vi "Is New State.vi"(8 "error in (no error)":errorcluster, 11 "Command in":refnum<class "Command.lvclass">) -> (0 "error out":errorcluster, 3 "Command out":refnum<class "Command.lvclass">)   [LabVIEW 2013, in "Command.lvclass"]
uses:
  Command.lvclass
  Command.lvclass/Command.ctl
  States/State/State.lvclass
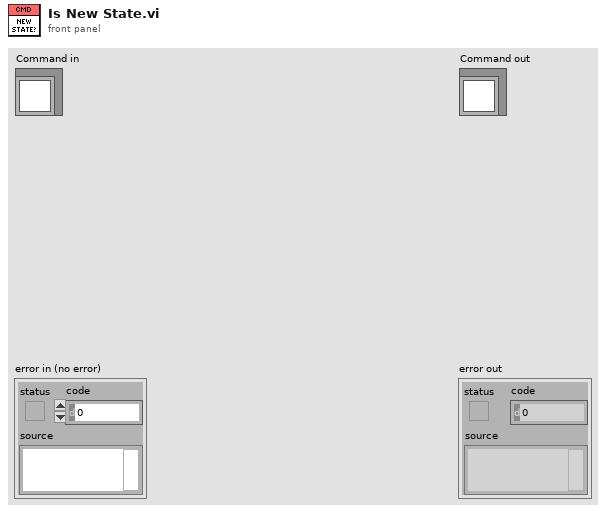
[diagram p1: front panel]
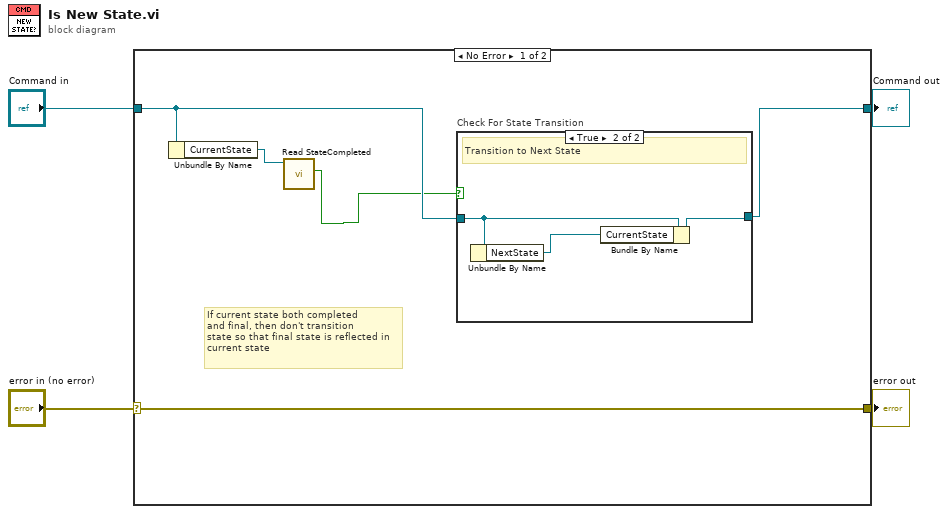
[diagram p0: block diagram]
diagram:
  n1 = case shown="No Error" "error in (no error)" {
    selector: "error in (no error)" -> [w9 w15]
    tunnel: [w9 w15] -> w3
    tunnel: [w6 w14] -> w1
    tunnel: "Command in" -> [w7 w14]
    frame No Error {
      # "If current state both completed\nand final, then don't transition \nstate so that final state is reflected in \ncurrent state"
      n2 = Unbundle By Name(w7) -> ("CurrentState"=w8:refnum<class "State.lvclass">)
      n3 = call-dynamic "Read StateCompleted.vi"("State in"=w8) -> ("StateCompleted"=w5:bool)  [unwired: 8 in, 2 out]
      n4 = case "Check For State Transition" shown="True" w5 {
        tunnel: [w10 w12] -> w6
        tunnel: w7 -> [w10 w13]
        frame False {
          # "No State Transition"
        }
        frame True {
          # "Transition to Next State"
          n5 = Unbundle By Name(w13) -> ("NextState"=w11:refnum<class "State.lvclass">)
          n6 = Bundle By Name(cluster=w13, "CurrentState"=w11) -> (w12:refnum<class "Command.lvclass">)
        }
      }
    }
    frame Error {
    }
  }
  "error out" <- w3
  "Command out" <- w1
